vi "DataToRead.vi"(8 "error in (no error)":errorcluster, 11 "TcpReader in":refnum<class "TcpReader.lvclass">) -> (0 "error out":errorcluster, 2 "Data available?":bool, 3 "TcpReader out":refnum<class "TcpReader.lvclass">)   [LabVIEW 2025, in "TcpReader.lvclass"]
doc: "Returns TRUE if there is any data to read from the remote host"
uses:
  TcpReader.lvclass
  TcpReader.lvclass/TcpReader.ctl
  <userlib>/_OpenG.lib/error/error.llb/Filter Error Codes (Array)__ogtk.vi
  Interface/TCP/TCP/TCP.lvclass
  <userlib>/_OpenG.lib/error/error.llb/openg_error.lvlib
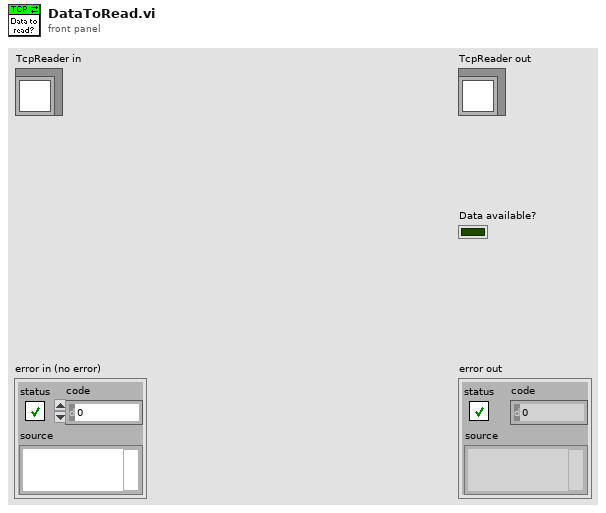
[diagram p1: front panel]
types:
  T1 = enum16{"Standard", "Buffered", "CRLF", "Immediate"}
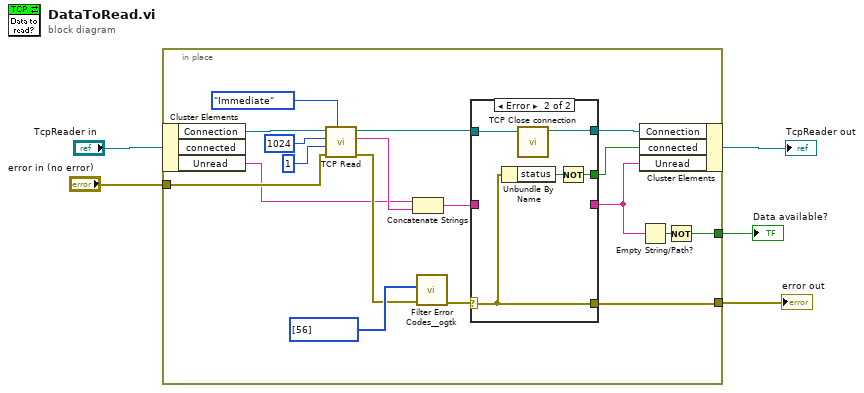
[diagram p0: block diagram]
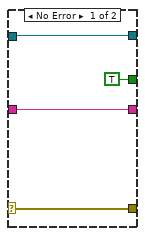
[diagram p2: hidden frame]
diagram:
  n1 = in-place "In Place Element Structure" {
    in-place-border: "error in (no error)" -> [w19]
    in-place-border: [w12] -> w3
    in-place-border: [w14] -> w2
    n2 = in-place-cluster #1("TcpReader in") -> ("Connection"=w23:refnum<class "TCP.lvclass">, "Unread"=w6:string)  [unwired: 1 out]
    n3 = call-dynamic "TCP Read.vi"("mode (standard)"=T1."Immediate", "error in (no error)"=w19, "timeout ms (25000)"=1, "bytes to read"=1024, "TCP in"=w23) -> ("error out"=w15:errorcluster, "data out"=w18:string, "TCP out"=w10:refnum<class "TCP.lvclass">)  [unwired: 4 in]
    n4 = Concatenate Strings(w6, w18) -> (w11:string)
    n5 = call-poly <userlib>:"Filter Error Codes__ogtk.vi"("Error In"=w15, "Error Codes to Filter"=i32[] [56]) -> ("Error Out"=w13:errorcluster)  [unwired: 7 in, 2 out]
    n6 = case shown="Error" w13 {
      selector: w13 -> [w26 w28]
      tunnel: w10 -> [w24 w32]
      tunnel: [w24 w31] -> w9
      tunnel: [TRUE w29] -> w8
      tunnel: [w26 w28] -> w12
      tunnel: [w25 _] -> w7
      tunnel: w11 -> [w25 _]
      frame No Error {
      }
      frame Error {
        n7 = Unbundle By Name(w28) -> ("status"=w30:bool)
        n8 = call-dynamic "TCP Close connection.vi"("TCP in"=w32) -> ("TCP out"=w31:refnum<class "TCP.lvclass">)  [unwired: 9 in, 1 out]
        n9 = Not(x=w30) -> (.not. x?=w29:bool)
      }
    }
    n10 = in-place-cluster #1("Connection"=w9, "connected"=w8, "Unread"=w7) -> (→"TcpReader out":refnum<class "TcpReader.lvclass">)
    n11 = Empty String/Path?(string/path=w7) -> (empty?=w17:bool)
    n12 = Not(x=w17) -> (.not. x?=w14:bool)
  }
  "error out" <- w3
  "Data available?" <- w2
